vi "While Loop Basics.vi"() -> ()   [LabVIEW 2019]
panel:
  out "Hours":dbl
  out "Minutes":dbl
  out "Seconds":dbl
  in  "Total Time in Seconds":dbl
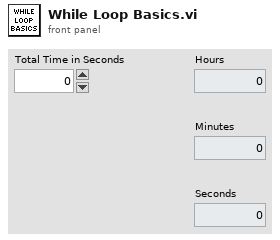
[diagram p1: front panel]
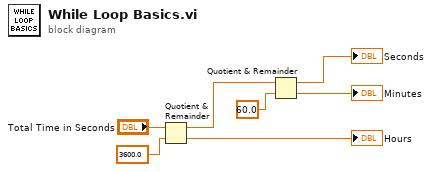
[diagram p0: block diagram]
diagram:
  n1 = Quotient & Remainder(x="Total Time in Seconds", y=3600.0) -> (x-y*floor(x/y)=w3:dbl, floor(x/y)=→"Hours":dbl)
  n2 = Quotient & Remainder(x=w3, y=60.0) -> (x-y*floor(x/y)=→"Seconds":dbl, floor(x/y)=→"Minutes":dbl)
